vi "makeTIUnderlayPlotCommands.vi"(6 "plotInfoArray":T1(array[cluster]), 9 "Scale":dbl=300.0 caption="Scale 1:" min=1.0 max=10000.0 step=50.0) -> (1 "UnderlayPlotSeries":string[](array[string]), 2 "Pre-plot Injection":string, 3 "Basics Visible":bool[](array[boolean]))   [LabVIEW 2021]
uses:
  at.ctl
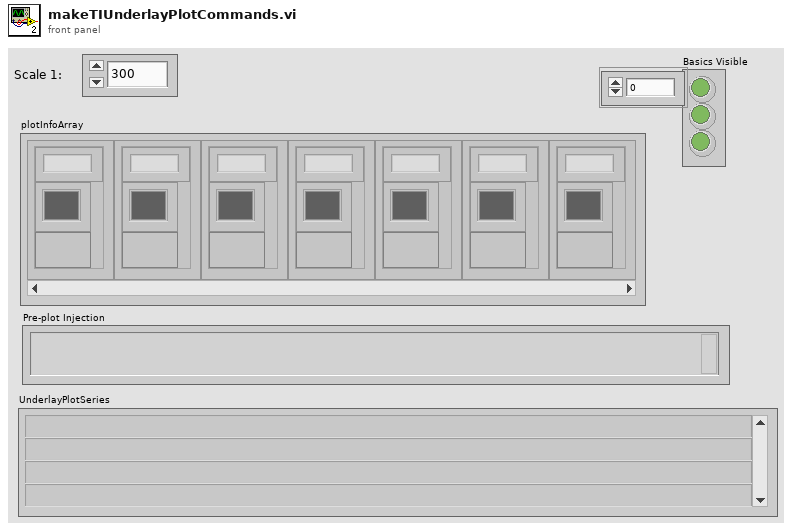
[diagram p1: front panel]
types:
  T1 = cluster{"Plot Name":string, "Plot.Plot Color":u32, "Plot.Visible?":bool}[]
  T2 = typedef "at.ctl" = cluster{"XcoordSys":string, "YcoordSys":string, "Xvalue":dbl, "Yvalue":dbl}
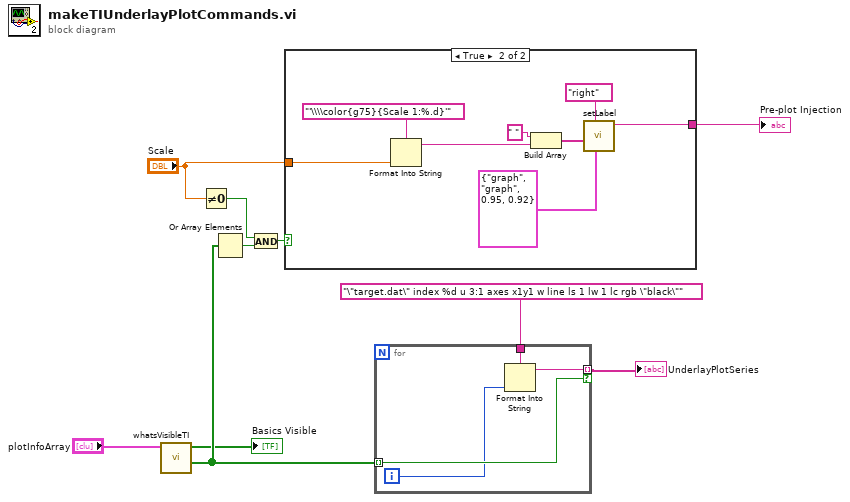
[diagram p0: block diagram]
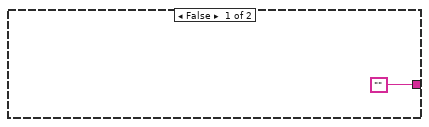
[diagram p2: hidden frame]
diagram:
  n1 = call "whatsVisibleTI.vi"("TIplotInfoArray"="plotInfoArray") -> ("Targets Visible"=w7:bool[], "Basics Visible"=→"Basics Visible":bool[])  [unwired: 9 in]
  n2 = Not Equal To 0?(x="Scale") -> (x != 0?=w1:bool)
  n3 = Or Array Elements(Boolean array=w7) -> (logical OR=w5:bool)
  n4 = And(x=w1, y=w5) -> (x .and. y?=w2:bool)
  n5 = case shown="True" w2 {
    tunnel: ["" w13] -> w6
    tunnel: "Scale" -> [_ w12]
    frame False {
    }
    frame True {
      n6 = Format Into String(format string="'\\\\color{g75}{Scale 1:%.d}'", w12) -> (resulting string=w19:string)  [unwired: 2 in, 1 out]
      n7 = Build Array(" " ("element"), w19) -> (w18:string[])
      n8 = call "setLabel.vi"("\"At\" location"=T2 {"XcoordSys"="graph", "YcoordSys"="graph", "Xvalue"=0.95, "Yvalue"=0.92} ("\"At\" location"), "Justify"="right", "multilineLabel"=w18) -> ("String out"=w13:string)  [unwired: 7 in, 1 out]
    }
  }
  "Pre-plot Injection" <- w6
  n9 = for {
    tunnel: [w23] -> w8 mode=indexing if=w22
    tunnel: w7 -> [w22] mode=indexing
    tunnel: "\"target.dat\" index %d u 3:1 axes x1y1 w line ls 1 lw 1 lc rgb \"black\"" ("String") -> [w21]
    i -> [w20]
    n10 = Format Into String(format string=w21, w20) -> (resulting string=w23:string)  [unwired: 2 in, 1 out]
  }
  "UnderlayPlotSeries" <- w8
